vi "Periodic Tasks.vi"(8 "error in":errorcluster) -> ()   [LabVIEW 2019]
doc: "This VI runs in parallel to other tasks. It can contain as many user-defined periodic loops as you need. These can carry out PID or other sorts of timed response."
uses:
  <vilib>/Rock Robotics/WPI/ThirdParty/JAS_Junk/TrajLib/VI/Util_GetTime_U32.vi
  <vilib>/Rock Robotics/WPI/ThirdParty/JAS_Junk/TrajLib/MathUtil_Clamp.vi
  <vilib>/Rock Robotics/WPI/ThirdParty/JAS_Junk/TrajLib/VI/Util_GetTime_U64.vi
  Robot Global Data.vi
  <vilib>/Rock Robotics/Network Tables/NT Write Number.vi
  <vilib>/Rock Robotics/WPI/ThirdParty/JAS_Junk/TrajLib/Trajectory_Library.lvlib
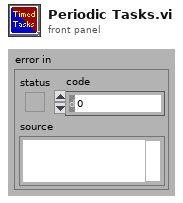
[diagram p1: front panel]
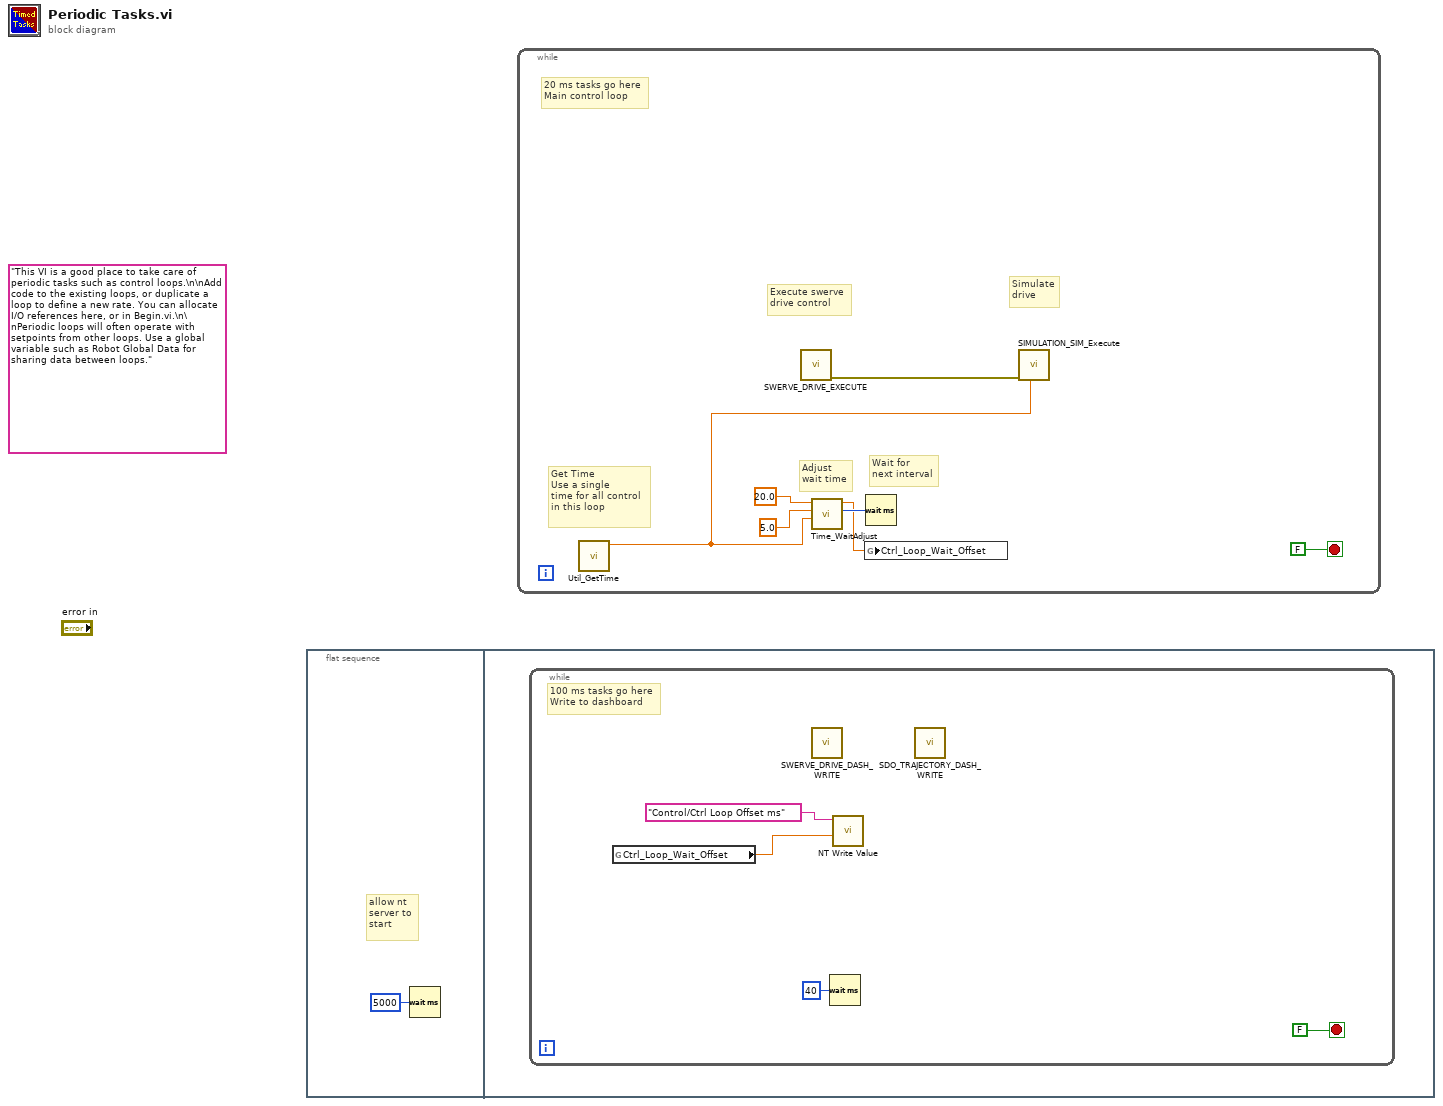
[diagram p0: block diagram]
diagram:
  (unwired) "This VI is a good place to take care of periodic tasks such as control loops.\n\nAdd code to the existing loops, or duplicate a loop to define a new rate. You can allocate I/O references here, or in Begin.vi.\n\nPeriodic loops will often operate with setpoints from other loops. Use a global variable such as Robot Global Data for sharing data between loops."
  n1 = flat-sequence {
    frame #0 {
      # "allow nt\nserver to \nstart"
      n2 = Wait (ms)(milliseconds to wait=u32 5000) -> ()  [unwired: 1 out]
    }
    frame #1 {
      n3 = while {
        stop <- FALSE stop-if-true
        # "100 ms tasks go here\nWrite to dashboard"
        n4 = global read "Robot Global Data.vi" "Ctrl_Loop_Wait_Offset"() -> (w2:dbl)
        n5 = call "SWERVE_DRIVE_DASH_WRITE.vi"() -> ()  [unwired: 12 in]
        n6 = Wait (ms)(milliseconds to wait=u32 40) -> ()  [unwired: 1 out]
        n7 = call-poly <vilib>:"NT Write Value.vi"("value"=w2, "name"="Control/Ctrl Loop Offset ms" ("Name")) -> ()  [unwired: 9 in, 1 out]
        n8 = call "SDO_TRAJECTORY_DASH_WRITE.vi"() -> ()  [unwired: 12 in]
      }
    }
  }
  n9 = while {
    stop <- FALSE stop-if-true
    # "Simulate\ndrive"
    # "Execute swerve\ndrive control"
    # "Wait for\nnext interval"
    # "Adjust\nwait time"
    # "Get Time\nUse a single\ntime for all control\nin this loop"
    # "20 ms tasks go here\nMain control loop"
    n10 = call <vilib>:"Util_GetTime.vi"() -> ("FPGA_Time_Seconds"=w7:dbl)  [unwired: 9 in, 2 out]
    n11 = call "SWERVE_DRIVE_EXECUTE.vi"() -> ("error out"=w6:errorcluster)  [unwired: 11 in]
    n12 = call <vilib>:"Time_WaitAdjust.vi"("PassthroughTime_SEC"=w7, "MaxAdjustment_MS"=5.0 ("MaxDeviation_MS"), "DesiredLoopTime_MS"=20.0) -> ("AdjustedWaitTime_MS"=w9:u32, "Offset_MS"=w8:dbl)  [unwired: 7 in]
    n13 = global write "Robot Global Data.vi" "Ctrl_Loop_Wait_Offset"(w8) -> ()
    n14 = Wait (ms)(milliseconds to wait=w9) -> ()  [unwired: 1 out]
    n15 = call "SIMULATION_SIM_Execute.vi"("FPGA_Time_Seconds"=w7, "error in (no error)"=w6) -> ()  [unwired: 9 in, 1 out]
  }
